vi "Get All PPLs Under Target.vi"(8 "error in (no error)":errorcluster, 10 "exclude dependencies (F)":bool, 11 "Target":refnum<vi>) -> (0 "error out":errorcluster, 2 "PPL Names":string[](array[string]), 3 "PPLs under target":refnum<vi>[](array[refnum]))   [LabVIEW 2020, in "AFPP Shared.lvlib"]
uses:
  AFPP Shared.lvlib
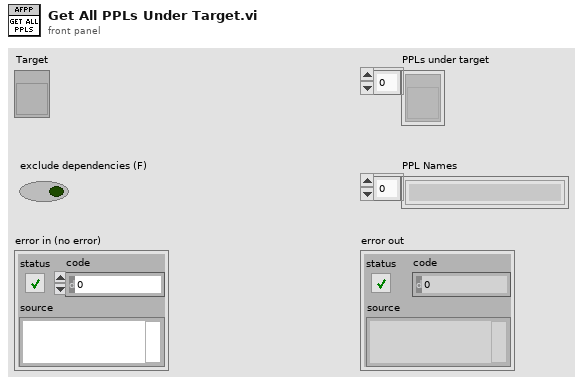
[diagram p1: front panel]
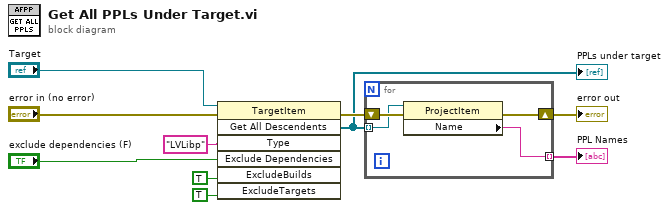
[diagram p0: block diagram]
diagram:
  n1 = invoke class="TargetItem" method="Get All Descendents"(reference="Target", error in="error in (no error)", "Type"="LVLibp", "Exclude Dependencies"="exclude dependencies (F)", "ExcludeBuilds"=TRUE, "ExcludeTargets"=TRUE) -> (error out=w5:errorcluster, "All Descendents"=w4:refnum<vi>[])  [unwired: 1 in, 5 out]
  "PPLs under target" <- w4
  n2 = for {
    shift-right: [w11] -> w2
    shift-left: w5 -> [w14]
    tunnel: w4 -> [w13] mode=indexing
    tunnel: [w12] -> w3 mode=indexing
    n3 = property class="ProjectItem"(reference=w13, error in=w14) -> (error out=w11:errorcluster, "Name"=w12:string)  [unwired: 1 out]
  }
  "PPL Names" <- w3
  "error out" <- w2
